vi "U1_E3_final.vi"() -> ()   [LabVIEW 2016]
panel:
  out "Error":bool
  in  "Divide":bool
  in  "Multiply":bool
  in  "Substract":bool
  out "Iteration":i32
  in  "stop":bool
  out "Result":dbl
  in  "Sum":bool
  in  "Number1":dbl
  in  "Number2":dbl
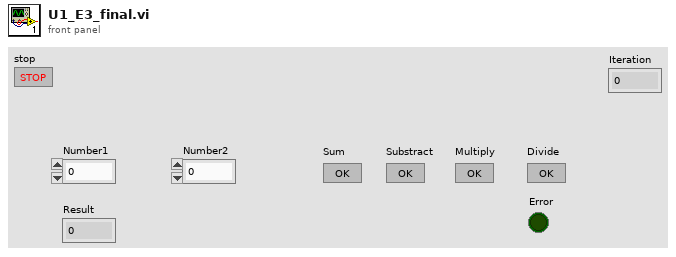
[diagram p1: front panel]
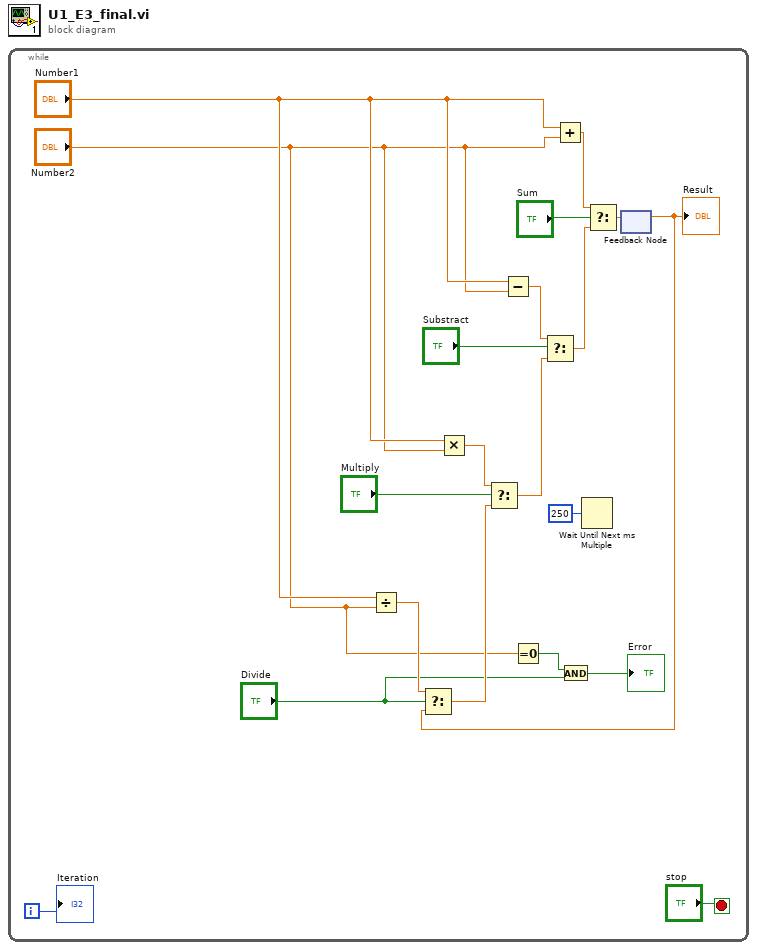
[diagram p0: block diagram]
diagram:
  n1 = while {
    i -> [w18]
    stop <- "stop" stop-if-true
    n2 = Divide(x="Number1", y="Number2") -> (x/y=w10:dbl)
    n3 = Multiply(x="Number1", y="Number2") -> (x*y=w14:dbl)
    n4 = Subtract(x="Number1", y="Number2") -> (x-y=w17:dbl)
    n5 = Equal To 0?(x="Number2") -> (x = 0?=w3:bool)
    n6 = Add(x="Number1", y="Number2") -> (x+y=w20:dbl)
    n7 = And(x=w3, y="Divide") -> (x .and. y?=→"Error":bool)
    n8 = Wait Until Next ms Multiple(millisecond multiple=u32 250) -> ()  [unwired: 1 out]
    n9 = feedback #1() -> (w11:dbl)  [unwired: 1 in]
    "Result" <- w11
    n10 = Select(t=w10, s="Divide", f=w11) -> (s? t:f=w9:dbl)
    n11 = Select(t=w14, s="Multiply", f=w9) -> (s? t:f=w15:dbl)
    n12 = Select(t=w17, s="Substract", f=w15) -> (s? t:f=w16:dbl)
    n13 = Select(t=w20, s="Sum", f=w16) -> (s? t:f=w12:dbl)
    n14 = feedback-in #1(w12) -> ()
    "Iteration" <- w18
  }
